vi "x_2.91_input.vi"() -> ()   [LabVIEW 2022 SP3]
panel:
  in  "gem og luk":bool
  in  "b":dbl
  in  "a":dbl=1.0
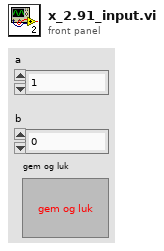
[diagram p1: front panel]
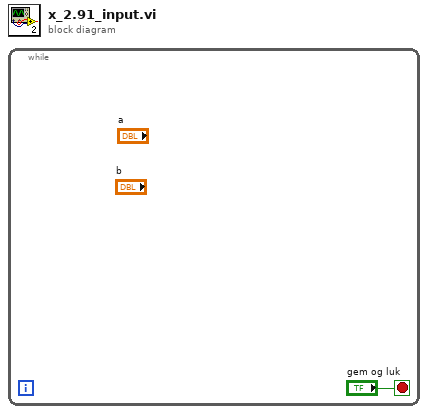
[diagram p0: block diagram]
diagram:
  n1 = while {
    stop <- "gem og luk" stop-if-true
  }
